vi "CRYSelect DAT&RES list.vi"(0 "Selected Data Item":string[](array[string]), 5 "Selected Result Item":string[](array[string]), 7 "Data Names":string[](array[string]), 9 "Result Names":string[](array[string])) -> (4 "Data Index":i32[](array[numeric]), 6 "Result Index":i32[](array[numeric]))   [LabVIEW 2013]
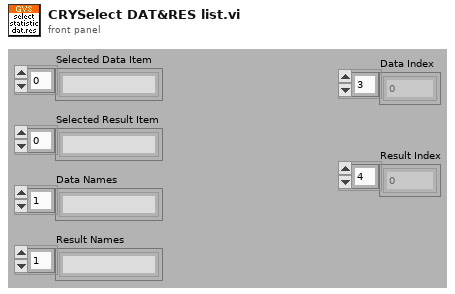
[diagram p1: front panel]
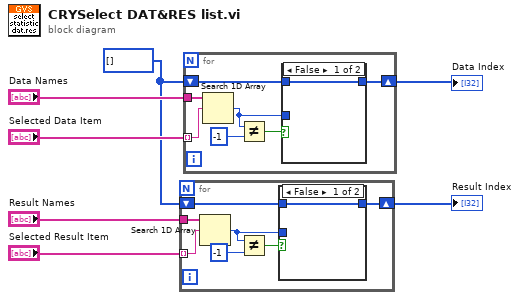
[diagram p0: block diagram]
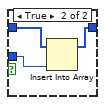
[diagram p2: hidden frame]
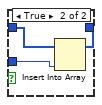
[diagram p3: hidden frame]
diagram:
  w2 = i32[] [] ("Data Index")
  n1 = for {
    tunnel: "Result Names" -> [w14]
    tunnel: "Selected Result Item" -> [w13] mode=indexing
    shift-right: [w8] -> w1
    shift-left: w2 -> [w9]
    n2 = Search 1D Array(1D array=w14, element=w13) -> (index of element=w10:i32)  [unwired: 1 out]
    n3 = Not Equal?(x=w10, y=-1) -> (x != y?=w11:bool)
    n4 = case shown="False" w11 {
      tunnel: w10 -> [_ w18]
      tunnel: w9 -> [w15 w17]
      tunnel: [w15 w16] -> w8
      frame False {
      }
      frame True {
        n5 = Insert Into Array(array=w17, new element=w18) -> (w16:i32[])  [unwired: 1 in]
      }
    }
  }
  "Result Index" <- w1
  n6 = for {
    tunnel: "Data Names" -> [w25]
    tunnel: "Selected Data Item" -> [w24] mode=indexing
    shift-right: [w19] -> w3
    shift-left: w2 -> [w20]
    n7 = Search 1D Array(1D array=w25, element=w24) -> (index of element=w21:i32)  [unwired: 1 out]
    n8 = Not Equal?(x=w21, y=-1) -> (x != y?=w22:bool)
    n9 = case shown="False" w22 {
      tunnel: w21 -> [_ w29]
      tunnel: w20 -> [w26 w28]
      tunnel: [w26 w27] -> w19
      frame False {
      }
      frame True {
        n10 = Insert Into Array(array=w28, new element=w29) -> (w27:i32[])  [unwired: 1 in]
      }
    }
  }
  "Data Index" <- w3
